vi "Subtract Background.vi"(8 "error in (no error)":errorcluster, 10 "Spectrum":dbl[](array[numeric]), 11 "Ocean Optics Driver in":refnum<class "Ocean Optics Driver.lvclass">) -> (0 "error out":errorcluster, 2 "Spectrum out":dbl[](array[numeric]), 3 "Ocean Optics Driver out":refnum<class "Ocean Optics Driver.lvclass">)   [LabVIEW 2016, in "Ocean Optics Driver.lvclass"]
uses:
  Ocean Optics Driver.lvclass
  Ocean Optics Driver.lvclass/Ocean Optics Driver.ctl
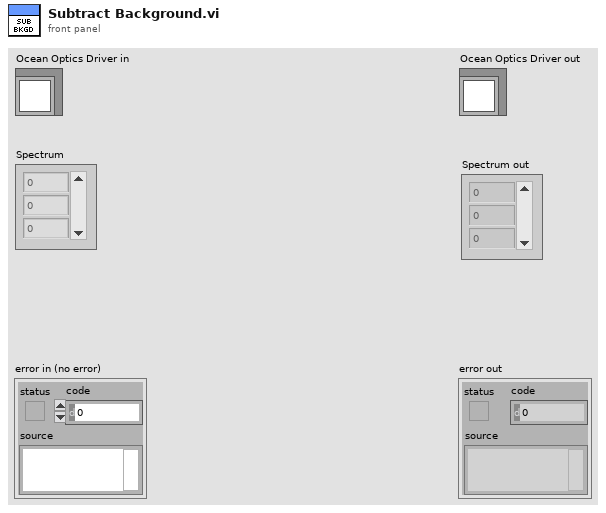
[diagram p1: front panel]
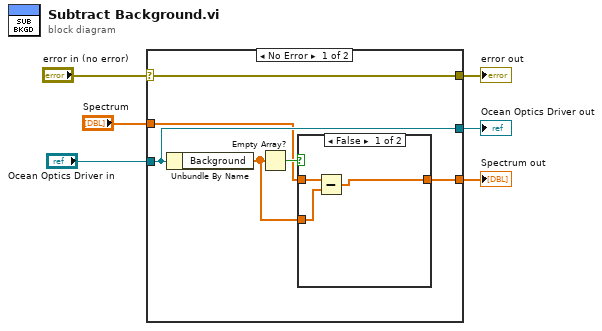
[diagram p0: block diagram]
diagram:
  n1 = case shown="No Error" "error in (no error)" {
    selector: "error in (no error)" -> [w12 w19]
    tunnel: [w12 w19] -> w5
    tunnel: [w11 w18] -> w3
    tunnel: "Ocean Optics Driver in" -> [w11 w18]
    tunnel: "Spectrum" -> [w9 w17]
    tunnel: [w8 w17] -> w1
    frame No Error {
      n2 = Unbundle By Name(w11) -> ("Background"=w7:dbl[])
      n3 = Empty Array?(array=w7) -> (empty?=w10:bool)
      n4 = case shown="False" w10 {
        tunnel: w9 -> [w14 w16]
        tunnel: [w13 w16] -> w8
        tunnel: w7 -> [w15 _]
        frame False {
          n5 = Subtract(x=w14, y=w15) -> (x-y=w13:dbl[])
        }
        frame True {
        }
      }
    }
    frame Error {
    }
  }
  "error out" <- w5
  "Ocean Optics Driver out" <- w3
  "Spectrum out" <- w1
